vi "Test_DL-EN1.vi"(8 "Fehler in":errorcluster, 9 "ID Messverstärker":u32=1 min=1 max=2, 10 "Befehl":T10, 11 "Cluster in":T2={"Initialisierung"={"Online?"=FALSE, "Grundpfad"=path "", "Kamera Oben"="", "IP-Adresse Flüssiglinse"="", "Flüssiglinse"=refnum, "Kamera Unten"="", "IP-Adresse SPS"="", "SPS-Verbindung"={"TCP Connection Ref"=refnum, "IP address"="", "timeout ms"=5000, "Connected?"=FALSE, "PLC Type"=enum."S7 1200", "Rack S7 400"=0, "Slot S7 400"=0, "PDU Size"=0, "connection semaphore"=refnum}, "IP-Adresse Lichtgitter"="", "Lichtgitter"=refnum, "Skalierungsfaktor"=0.0, "Bilder Oben"=[], "Bild Unten"=refnum, "Bild Ausschnitt Unten"=refnum}, "Einstellungen"={"Gesamtablauf gestartet"=FALSE, "i. O. Bilder speichern"=FALSE, "Bildspeicherung Offline"=FALSE, "Ausgewähltes Offline-Datum"="", "Ausgewähltes Offline-Teil"="", "Speicherpfad Bilder"=path ""}, "Artikeldaten"={"Artikelnummer"="", "Fertigungsauftrag"="", "Muster ISO"=refnum, "Belichtungszeit Referenzmarken"=0.0, "Fokus Referenzmarken"=0.0, "Belichtungszeit ISO"=0.0, "Fokus ISO"=0.0, "Belichtungszeit Unten"=0.0, "Kontaktanzahl"=0, "Aktueller Kontakt"=0, "Kontaktposition"={"x"=0.0, "y"=0.0}, "Winkel ISO"=0.0, "ISO-Muster nicht vorhanden"=FALSE}, "Werte Kamera Oben"={"Koordinatensystem"={"Punkt x-Achse"={"X"=0.0, "Y"=0.0}, "Ursprung"={"X"=0.0, "Y"=0.0}, "Punkt y-Achse"={"X"=0.0, "Y"=0.0}}, "Position Kontakt"={"x"=0.0, "y"=0.0}, "Winkel Kontakt"=0.0}, "Werte Kamera Unten"={"Prüfung Unten n. i. O."=FALSE}, "Werte Lichtgitter"={"Messwerte Referenzmarken"=[], "Mittelpunkt Referenzmarken"={"x"=0.0, "y"=0.0}, "Messwerte Kontakt"=[], "Offset"={"x"=0.0, "y"=0.0}}, "Rückmeldungen"={"Koordinaten ermittelt"=FALSE, "Vermessung Lichtgitter fertig"=FALSE, "Nachkontrolle Kamera Unten fertig"=FALSE}, "Fehler"={"Referenzen nicht gefunden"=FALSE, "Kontakt nicht gefunden"=FALSE, "Referenzen nicht in Lichtgitter"=FALSE, "Kontakt zu groß"=FALSE, "Kontakt zu klein"=FALSE}, "Statistik"={"Statistiken"=[]}, "Timer"={"Timer Start Position"=0, "Timer Start Lichtgitter"=0, "Timer Start Kamera Unten"=0}}) -> (0 "Fehler out":errorcluster, 1 "Lese- und Schreibestrings":string, 2 "Lichtgitter Cluster out":T1, 3 "Cluster out":T2={"Initialisierung"={"Online?"=FALSE, "Grundpfad"=path "", "Kamera Oben"="", "IP-Adresse Flüssiglinse"="", "Flüssiglinse"=refnum, "Kamera Unten"="", "IP-Adresse SPS"="", "SPS-Verbindung"={"TCP Connection Ref"=refnum, "IP address"="", "timeout ms"=5000, "Connected?"=FALSE, "PLC Type"=enum."S7 1200", "Rack S7 400"=0, "Slot S7 400"=0, "PDU Size"=0, "connection semaphore"=refnum}, "IP-Adresse Lichtgitter"="", "Lichtgitter"=refnum, "Skalierungsfaktor"=0.0, "Bilder Oben"=[], "Bild Unten"=refnum, "Bild Ausschnitt Unten"=refnum}, "Einstellungen"={"Gesamtablauf gestartet"=FALSE, "i. O. Bilder speichern"=FALSE, "Bildspeicherung Offline"=FALSE, "Ausgewähltes Offline-Datum"="", "Ausgewähltes Offline-Teil"="", "Speicherpfad Bilder"=path ""}, "Artikeldaten"={"Artikelnummer"="", "Fertigungsauftrag"="", "Muster ISO"=refnum, "Belichtungszeit Referenzmarken"=0.0, "Fokus Referenzmarken"=0.0, "Belichtungszeit ISO"=0.0, "Fokus ISO"=0.0, "Belichtungszeit Unten"=0.0, "Kontaktanzahl"=0, "Aktueller Kontakt"=0, "Kontaktposition"={"x"=0.0, "y"=0.0}, "Winkel ISO"=0.0, "ISO-Muster nicht vorhanden"=FALSE}, "Werte Kamera Oben"={"Koordinatensystem"={"Punkt x-Achse"={"X"=0.0, "Y"=0.0}, "Ursprung"={"X"=0.0, "Y"=0.0}, "Punkt y-Achse"={"X"=0.0, "Y"=0.0}}, "Position Kontakt"={"x"=0.0, "y"=0.0}, "Winkel Kontakt"=0.0}, "Werte Kamera Unten"={"Prüfung Unten n. i. O."=FALSE}, "Werte Lichtgitter"={"Messwerte Referenzmarken"=[], "Mittelpunkt Referenzmarken"={"x"=0.0, "y"=0.0}, "Messwerte Kontakt"=[], "Offset"={"x"=0.0, "y"=0.0}}, "Rückmeldungen"={"Koordinaten ermittelt"=FALSE, "Vermessung Lichtgitter fertig"=FALSE, "Nachkontrolle Kamera Unten fertig"=FALSE}, "Fehler"={"Referenzen nicht gefunden"=FALSE, "Kontakt nicht gefunden"=FALSE, "Referenzen nicht in Lichtgitter"=FALSE, "Kontakt zu groß"=FALSE, "Kontakt zu klein"=FALSE}, "Statistik"={"Statistiken"=[]}, "Timer"={"Timer Start Position"=0, "Timer Start Lichtgitter"=0, "Timer Start Kamera Unten"=0}})   [LabVIEW 2024]
doc: "Sendet den unter \"Befehl\" angegebenen Befehl an den Messverstärker der Lichtgitter und gibt dessen Antwort aus."
uses:
  Befehl_Lichtgitter.ctl
  Cluster.ctl
  Kontaktmontagemodul.exe/1abvi3w/vi.lib/userDefined/High Color/IMAQdx.ctl
  Kontaktmontagemodul.exe/1abvi3w/vi.lib/DATA AHEAD/SP7/typedefs/S7 Connection.ctl
  Kontaktmontagemodul.exe/1abvi3w/vi.lib/DATA AHEAD/SP7/typedefs/PLC Type.ctl
  Kontaktmontagemodul.exe/1abvi3w/vi.lib/vision/Image Controls.llb/IMAQ Image.ctl
  Koordinatensystem.ctl
  Statistik.ctl
  Cluster_out_Lichtgitter.ctl
  Kontaktmontagemodul.exe/1abvi3w/vi.lib/DATA AHEAD/SP7/SP7.lvlib
panel:
  out "Zeit alle Kanten in ms":u32
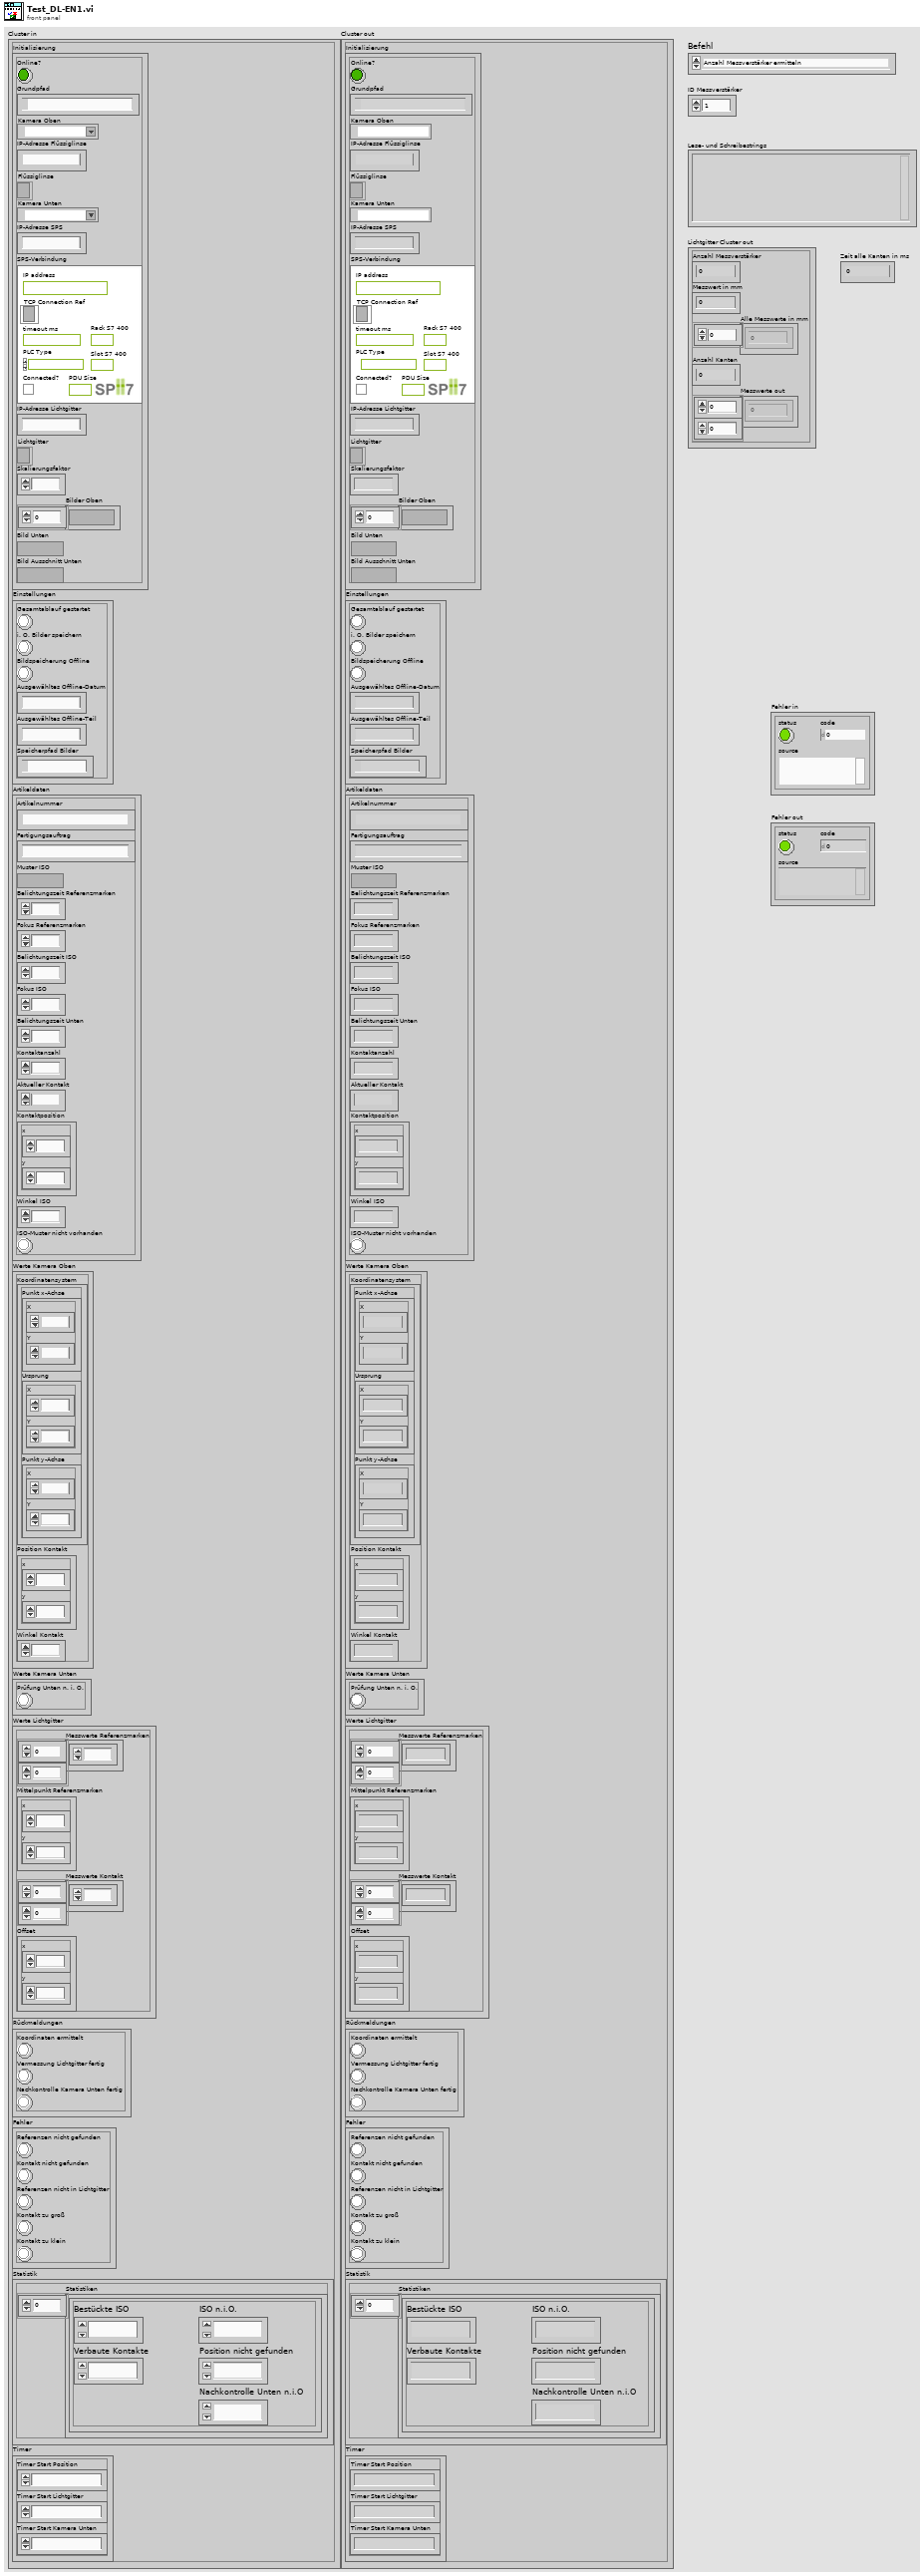
[diagram p1: front panel]
types:
  T1 = typedef "Cluster_out_Lichtgitter.ctl" = cluster{"Anzahl Messverstärker":i32, "Messwert in mm":dbl, "Alle Messwerte in mm":dbl[], "Anzahl Kanten":i32, "Messwerte out":dbl[][]}
  T2 = typedef "Cluster.ctl" = cluster{"Initialisierung":cluster{"Online?":bool, "Grundpfad":path, "Kamera Oben":T3, "IP-Adresse Flüssiglinse":string, "Flüssiglinse":refnum<k5>, "Kamera Unten":T3, "IP-Adresse SPS":string, "SPS-Verbindung":T4, "IP-Adresse Lichtgitter":string, "Lichtgitter":refnum<k5>, "Skalierungsfaktor":dbl, "Bilder Oben":T7[], "Bild Unten":T7, "Bild Ausschnitt Unten":T7}, "Einstellungen":cluster{"Gesamtablauf gestartet":bool, "i. O. Bilder speichern":bool, "Bildspeicherung Offline":bool, "Ausgewähltes Offline-Datum":string, "Ausgewähltes Offline-Teil":string, "Speicherpfad Bilder":path}, "Artikeldaten":cluster{"Artikelnummer":string, "Fertigungsauftrag":string, "Muster ISO":T7, "Belichtungszeit Referenzmarken":dbl, "Fokus Referenzmarken":dbl, "Belichtungszeit ISO":dbl, "Fokus ISO":dbl, "Belichtungszeit Unten":dbl, "Kontaktanzahl":u32, "Aktueller Kontakt":i16, "Kontaktposition":cluster{"x":sgl, "y":sgl}, "Winkel ISO":sgl, "ISO-Muster nicht vorhanden":bool}, "Werte Kamera Oben":cluster{"Koordinatensystem":T8, "Position Kontakt":cluster{"x":dbl, "y":dbl}, "Winkel Kontakt":dbl}, "Werte Kamera Unten":cluster{"Prüfung Unten n. i. O.":bool}, "Werte Lichtgitter":cluster{"Messwerte Referenzmarken":dbl[][], "Mittelpunkt Referenzmarken":cluster{"x":dbl, "y":dbl}, "Messwerte Kontakt":dbl[][], "Offset":cluster{"x":dbl, "y":dbl}}, "Rückmeldungen":cluster{"Koordinaten ermittelt":bool, "Vermessung Lichtgitter fertig":bool, "Nachkontrolle Kamera Unten fertig":bool}, "Fehler":cluster{"Referenzen nicht gefunden":bool, "Kontakt nicht gefunden":bool, "Referenzen nicht in Lichtgitter":bool, "Kontakt zu groß":bool, "Kontakt zu klein":bool}, "Statistik":cluster{"Statistiken":T9[]}, "Timer":cluster{"Timer Start Position":u32, "Timer Start Lichtgitter":u32, "Timer Start Kamera Unten":u32}}
  T3 = typedef "IMAQdx.ctl" = refnum<k21>
  T4 = typedef "SP7.lvlib/S7 Connection.ctl" = cluster{"TCP Connection Ref":refnum<k5>, "IP address":string, "timeout ms":i32, "Connected?":bool, "PLC Type":T5, "Rack S7 400":u8, "Slot S7 400":u8, "PDU Size":u16, "connection semaphore":T6}
  T5 = typedef "SP7.lvlib/PLC Type.ctl" = enum16{"S7 200", "S7 300/400", "S7 1200", "S7 1500", "LOGO!8"}
  T6 = typedef "Semaphore RefNum" = refnum<k1>
  T7 = typedef "IMAQ Image.ctl" = refnum<image>
  T8 = typedef "Koordinatensystem.ctl" = cluster{"Punkt x-Achse":cluster{"X":sgl, "Y":sgl}, "Ursprung":cluster{"X":sgl, "Y":sgl}, "Punkt y-Achse":cluster{"X":sgl, "Y":sgl}}
  T9 = typedef "Statistik.ctl" = cluster{"Bestückte ISO":u32, "Verbaute Kontakte":u32, "ISO n.i.O.":u32, "Nachkontrolle Unten n.i.O":u32, "Position nicht gefunden":u32}
  T10 = typedef "Befehl_Lichtgitter.ctl" = enum16{"Anzahl Messverstärker ermitteln", "Aktuellen Messwert von einem Messverstärker lesen", "Aktuellen Messwerte von allen Messverstärkern lesen", "Anzahl Kanten von einem Messverstärker ermitteln", "Alle Kanten von allen Messverstärkern lesen"}
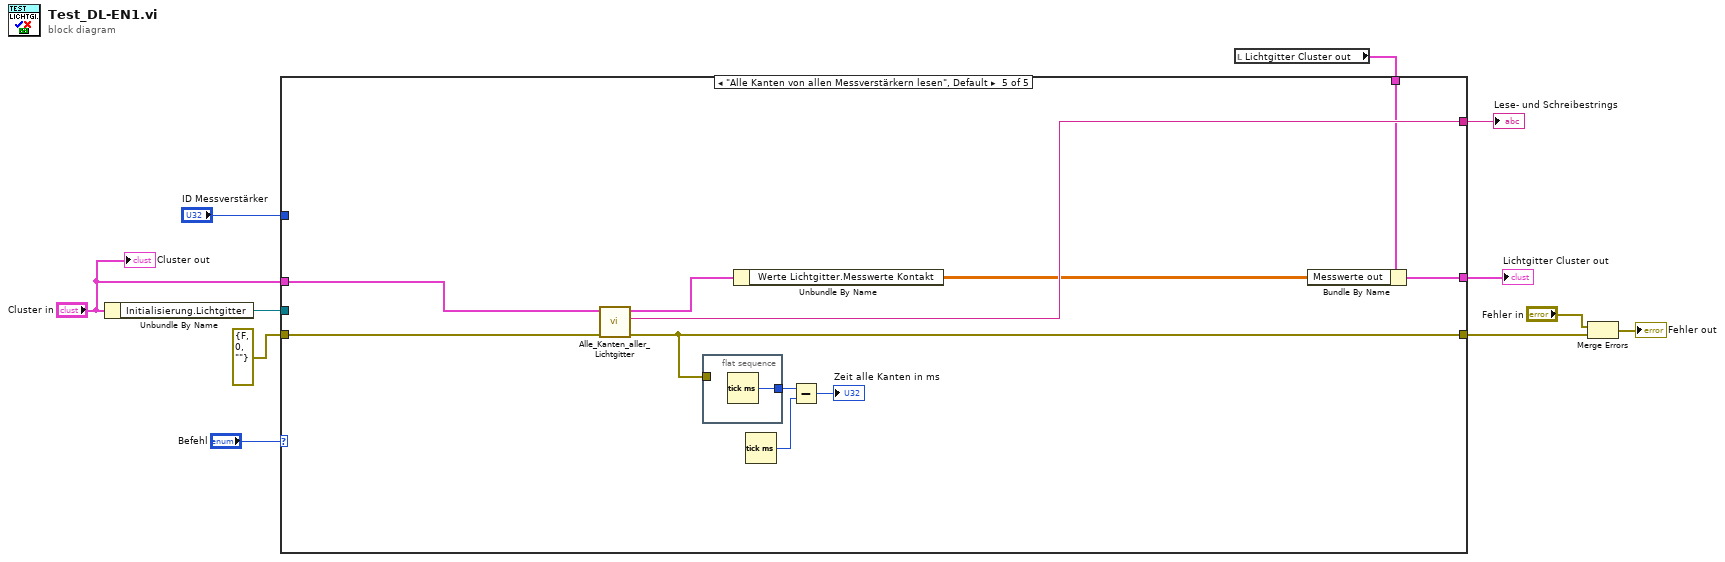
[diagram p0: block diagram]
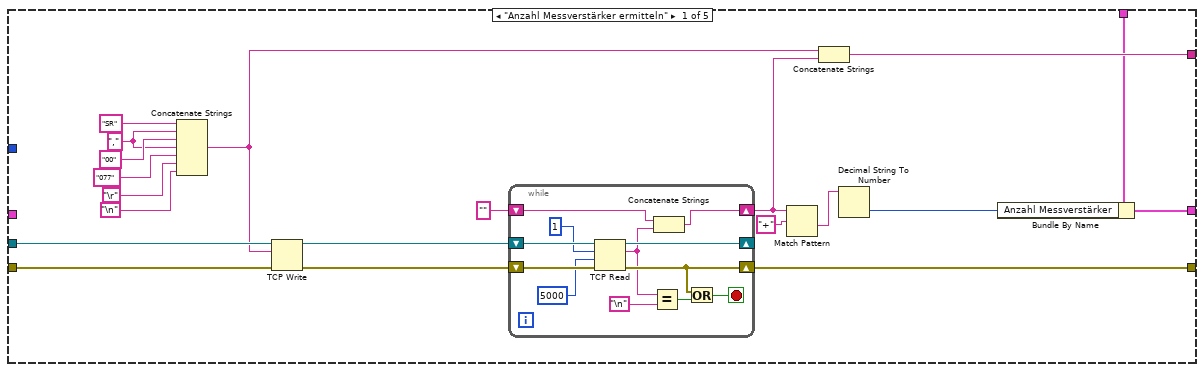
[diagram p2: hidden frame]
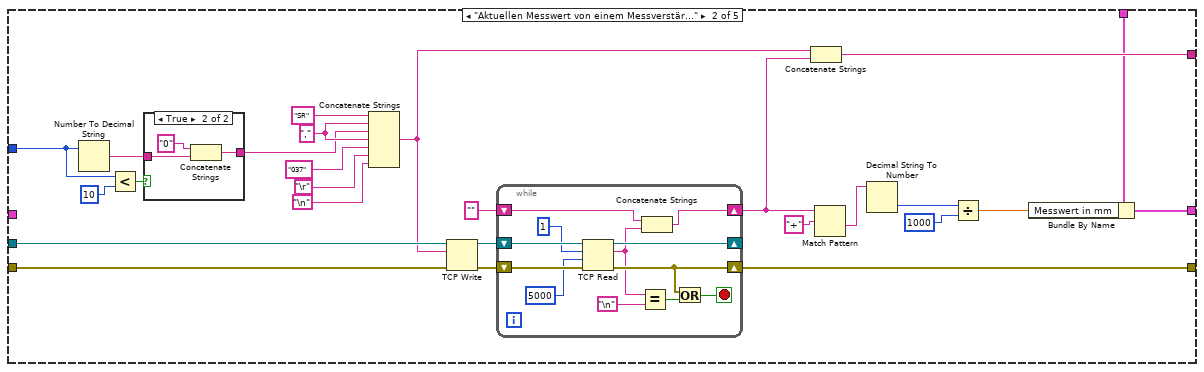
[diagram p3: hidden frame]
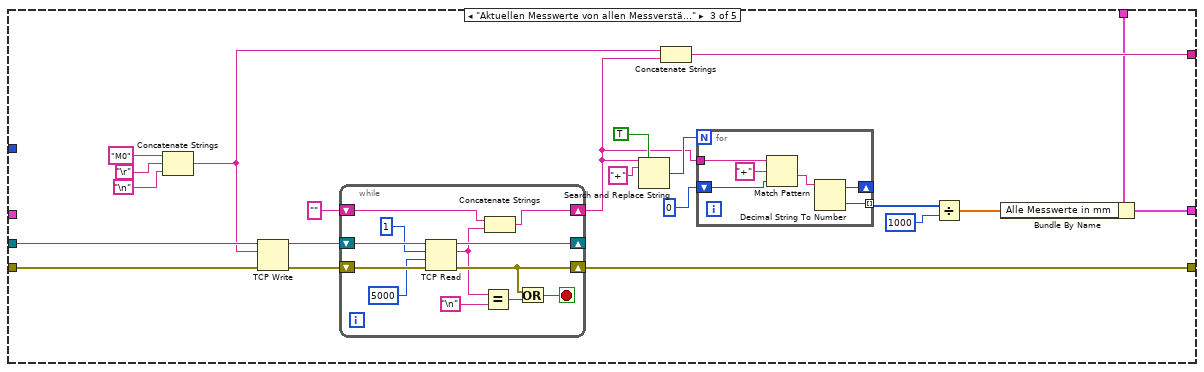
[diagram p5: hidden frame]
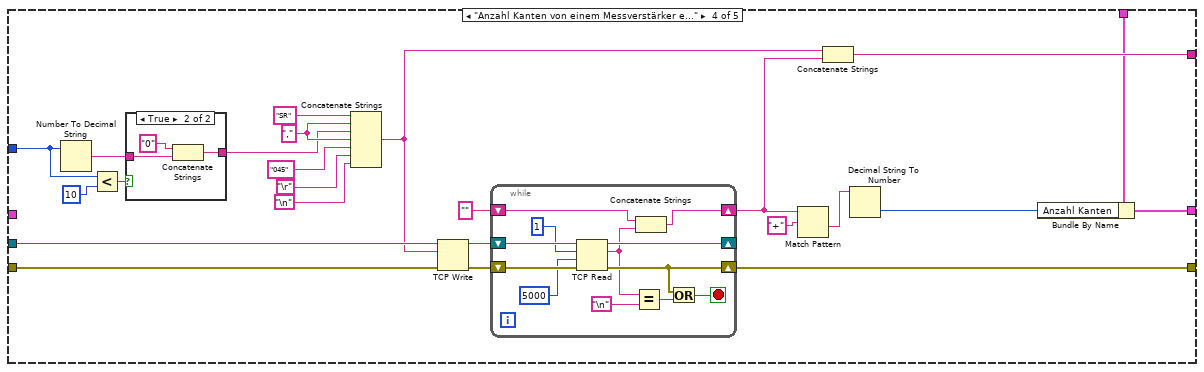
[diagram p6: hidden frame]
diagram:
  n1 = Unbundle By Name("Cluster in") -> ("Initialisierung.Lichtgitter"=w8:refnum<k5>)
  n2 = local read "Lichtgitter Cluster out"() -> (w1:T1)
  n3 = case shown="\"Alle Kanten von allen Messverstärkern lesen\", Default" "Befehl" {
    tunnel: errorcluster {"status"=FALSE, "code"=0, "source"=""} ("Fehler in") -> [w31 w60 w100 w144 w171]
    tunnel: w8 -> [w30 w61 w101 w145 _]
    tunnel: [w26 w59 w98 w143 w170] -> w5
    tunnel: [w15 w47 w89 w128 w169] -> w10
    tunnel: "ID Messverstärker" -> [_ w54 _ w133 _]
    tunnel: "Cluster in" -> [_ _ _ _ w172]
    tunnel: [w13 w44 w86 w125 w165] -> w2
    tunnel: w1 -> [w12 w46 w87 w126 w166]
    frame "Anzahl Messverstärker ermitteln" {
      w23 = "," ("string")
      n4 = Concatenate Strings("SR" ("data in"), w23, "00" ("string"), w23, "077" ("string"), "\r", "\n") -> (w17:string)
      n5 = TCP Write(connection ID=w30, data in=w17, error in (no error)=w31) -> (connection ID out=w28:refnum<k5>, error out=w27:errorcluster)  [unwired: 1 in, 1 out]
      n6 = while {
        shift-right: [w41] -> _
        shift-left: w28 -> [w43]
        shift-right: [w35] -> w26
        shift-left: w27 -> [w42]
        shift-right: [w38] -> w16
        shift-left: "" ("string") -> [w39]
        stop <- w34 stop-if-true
        n7 = TCP Read(connection ID=w43, bytes to read=1, error in (no error)=w42, 9:5000 ("timeout ms (25000)")) -> (connection ID out=w41:refnum<k5>, data out=w33:string, error out=w35:errorcluster)  [unwired: 1 in]
        n8 = Equal?(x=w33, y="\n") -> (x = y?=w36:bool)
        n9 = Concatenate Strings(w39, w33) -> (w38:string)
        n10 = Or(x=w35, y=w36) -> (x .or. y?=w34:bool)
      }
      n11 = Match Pattern(string=w16, regular expression="+") -> (after substring=w18:string)  [unwired: 1 in, 3 out]
      n12 = Concatenate Strings(w17, w16) -> (w15:string)
      n13 = Decimal String To Number(string=w18) -> (number=w14:i32)  [unwired: 2 in, 1 out]
      n14 = Bundle By Name(cluster=w12, "Anzahl Messverstärker"=w14) -> (w13:T1)
    }
    frame "Aktuellen Messwert von einem Messverstärker lesen" {
      w65 = "," ("string")
      n15 = Number To Decimal String(number=w54) -> (decimal integer string=w56:string)  [unwired: 1 in]
      n16 = Less?(x=w54, y=u32 10) -> (x < y?=w58:bool)
      n17 = case shown="True" w58 {
        tunnel: w56 -> [w70 w73]
        tunnel: [w70 w71] -> w55
        frame False {
        }
        frame True {
          n18 = Concatenate Strings("0" ("string"), w73) -> (w71:string)
        }
      }
      n19 = Concatenate Strings("SR" ("data in"), w65, w55, w65, "037" ("string"), "\r", "\n") -> (w49:string)
      n20 = TCP Write(connection ID=w61, data in=w49, error in (no error)=w60) -> (connection ID out=w68:refnum<k5>, error out=w67:errorcluster)  [unwired: 1 in, 1 out]
      n21 = while {
        shift-right: [w83] -> _
        shift-left: w68 -> [w85]
        shift-right: [w77] -> w59
        shift-left: w67 -> [w84]
        shift-right: [w80] -> w48
        shift-left: "" ("string") -> [w81]
        stop <- w76 stop-if-true
        n22 = TCP Read(connection ID=w85, bytes to read=1, error in (no error)=w84, 9:5000 ("timeout ms (25000)")) -> (connection ID out=w83:refnum<k5>, data out=w75:string, error out=w77:errorcluster)  [unwired: 1 in]
        n23 = Equal?(x=w75, y="\n") -> (x = y?=w78:bool)
        n24 = Concatenate Strings(w81, w75) -> (w80:string)
        n25 = Or(x=w77, y=w78) -> (x .or. y?=w76:bool)
      }
      n26 = Concatenate Strings(w49, w48) -> (w47:string)
      n27 = Match Pattern(string=w48, regular expression="+") -> (after substring=w52:string)  [unwired: 1 in, 3 out]
      n28 = Decimal String To Number(string=w52) -> (number=w51:i32)  [unwired: 2 in, 1 out]
      n29 = Divide(x=w51, y=1000) -> (x/y=w45:dbl)
      n30 = Bundle By Name(cluster=w46, "Messwert in mm"=w45) -> (w44:T1)
    }
    frame "Aktuellen Messwerte von allen Messverstärkern lesen" {
      n31 = Concatenate Strings("M0" ("data in"), "\r", "\n") -> (w91:string)
      n32 = TCP Write(connection ID=w101, data in=w91, error in (no error)=w100) -> (connection ID out=w106:refnum<k5>, error out=w105:errorcluster)  [unwired: 1 in, 1 out]
      n33 = while {
        shift-right: [w122] -> _
        shift-left: w106 -> [w124]
        shift-right: [w116] -> w98
        shift-left: w105 -> [w123]
        shift-right: [w119] -> w90
        shift-left: "" ("string") -> [w120]
        stop <- w115 stop-if-true
        n34 = TCP Read(connection ID=w124, bytes to read=1, error in (no error)=w123, 9:5000 ("timeout ms (25000)")) -> (connection ID out=w122:refnum<k5>, data out=w114:string, error out=w116:errorcluster)  [unwired: 1 in]
        n35 = Equal?(x=w114, y="\n") -> (x = y?=w117:bool)
        n36 = Concatenate Strings(w120, w114) -> (w119:string)
        n37 = Or(x=w116, y=w117) -> (x .or. y?=w115:bool)
      }
      n38 = Search and Replace String(replace all?=TRUE ("replace all? (F)"), input string=w90, search string="+") -> (number of replacements=w95:i32)  [unwired: 5 in, 3 out]
      n39 = Concatenate Strings(w91, w90) -> (w89:string)
      n40 = for {
        N: w95 -> [_]
        tunnel: w90 -> [w112]
        tunnel: [w109] -> w92 mode=indexing
        shift-right: [w108] -> _
        shift-left: 0 ("offset past number") -> [w107]
        n41 = Match Pattern(string=w112, regular expression="+" ("search string"), offset (0)=w107) -> (after substring=w110:string)  [unwired: 3 out]
        n42 = Decimal String To Number(string=w110) -> (offset past number=w108:i32, number=w109:i32)  [unwired: 2 in]
      }
      n43 = Divide(x=w92, y=1000) -> (x/y=w88:dbl[])
      n44 = Bundle By Name(cluster=w87, "Alle Messwerte in mm"=w88) -> (w86:T1)
    }
    frame "Anzahl Kanten von einem Messverstärker ermitteln" {
      w141 = "," ("string")
      n45 = Number To Decimal String(number=w133) -> (decimal integer string=w135:string)  [unwired: 1 in]
      n46 = Less?(x=w133, y=u32 10) -> (x < y?=w137:bool)
      n47 = case shown="True" w137 {
        tunnel: w135 -> [w149 w152]
        tunnel: [w149 w150] -> w134
        frame False {
        }
        frame True {
          n48 = Concatenate Strings("0" ("string"), w152) -> (w150:string)
        }
      }
      n49 = Concatenate Strings("SR" ("data in"), w141, w134, w141, "045" ("string"), "\r", "\n") -> (w130:string)
      n50 = TCP Write(connection ID=w145, data in=w130, error in (no error)=w144) -> (connection ID out=w148:refnum<k5>, error out=w147:errorcluster)  [unwired: 1 in, 1 out]
      n51 = while {
        shift-right: [w162] -> _
        shift-left: w148 -> [w164]
        shift-right: [w156] -> w143
        shift-left: w147 -> [w163]
        shift-right: [w159] -> w129
        shift-left: "" ("string") -> [w160]
        stop <- w155 stop-if-true
        n52 = TCP Read(connection ID=w164, bytes to read=1, error in (no error)=w163, 9:5000 ("timeout ms (25000)")) -> (connection ID out=w162:refnum<k5>, data out=w154:string, error out=w156:errorcluster)  [unwired: 1 in]
        n53 = Equal?(x=w154, y="\n") -> (x = y?=w157:bool)
        n54 = Concatenate Strings(w160, w154) -> (w159:string)
        n55 = Or(x=w156, y=w157) -> (x .or. y?=w155:bool)
      }
      n56 = Match Pattern(string=w129, regular expression="+") -> (after substring=w131:string)  [unwired: 1 in, 3 out]
      n57 = Concatenate Strings(w130, w129) -> (w128:string)
      n58 = Decimal String To Number(string=w131) -> (number=w127:i32)  [unwired: 2 in, 1 out]
      n59 = Bundle By Name(cluster=w126, "Anzahl Kanten"=w127) -> (w125:T1)
    }
    frame "Alle Kanten von allen Messverstärkern lesen", Default {
      n60 = call "Alle_Kanten_aller_Lichtgitter.vi"("Fehler in"=w171, "Cluster in"=w172) -> ("Fehler out"=w170:errorcluster, "Lese- und Schreibestrings"=w169:string, "Cluster out"=w168:T2)  [unwired: 6 in, 1 out]
      n61 = flat-sequence {
        tunnel: [w176] -> w175
        tunnel: w170 -> [_]
        frame #0 {
          n62 = Tick Count (ms)() -> (millisecond timer value=w176:u32)
        }
      }
      n63 = Unbundle By Name(w168) -> ("Werte Lichtgitter.Messwerte Kontakt"=w167:dbl[][])
      n64 = Tick Count (ms)() -> (millisecond timer value=w174:u32)
      n65 = Subtract(x=w175, y=w174) -> (x-y=→"Zeit alle Kanten in ms":u32)
      n66 = Bundle By Name(cluster=w166, "Messwerte out"=w167) -> (w165:T1)
    }
  }
  "Lese- und Schreibestrings" <- w10
  "Lichtgitter Cluster out" <- w2
  n67 = Merge Errors("Fehler in", w5) -> (→"Fehler out":errorcluster)
  "Cluster out" <- "Cluster in"
